vi "选择结构（求一个数的平方根）.vi"() -> ()   [LabVIEW 2017]
panel:
  out "平方根":dbl
  in  "输入":dbl
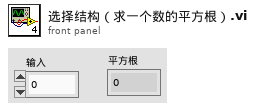
[diagram p1: front panel]
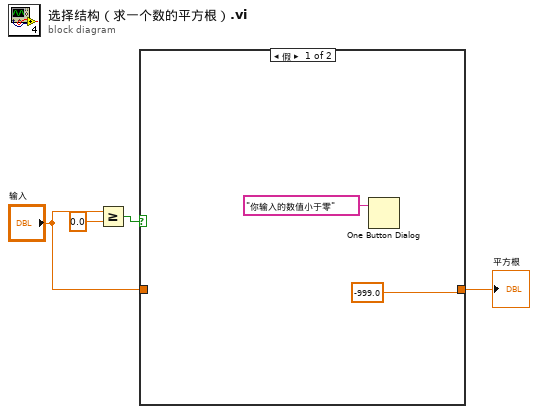
[diagram p0: block diagram]
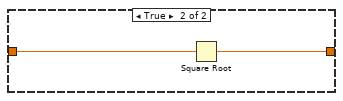
[diagram p2: hidden frame]
diagram:
  n1 = Greater Or Equal?(x="输入", y=0.0) -> (x >= y?=w3:bool)
  n2 = case shown="假" w3 {
    tunnel: "输入" -> [_ w8]
    tunnel: [-999.0 ("y") w7] -> w1
    frame False {
      n3 = One Button Dialog(message="你输入的数值小于零" ("消息")) -> ()  [unwired: 1 in, 1 out]
    }
    frame True {
      n4 = Square Root(x=w8) -> (sqrt(x)=w7:dbl)
    }
  }
  "平方根" <- w1
